vi "数据合并程序.vi"(8 "Save Files":path, 9 "File B":path, 10 "File A":path, 11 "File Item":path) -> ()   [LabVIEW 2011]
uses:
  <vilib>/Utility/file.llb/Read From Spreadsheet File (string).vi
  <vilib>/Utility/file.llb/Write To Spreadsheet File (string).vi
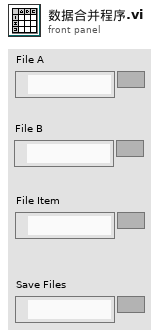
[diagram p1: front panel]
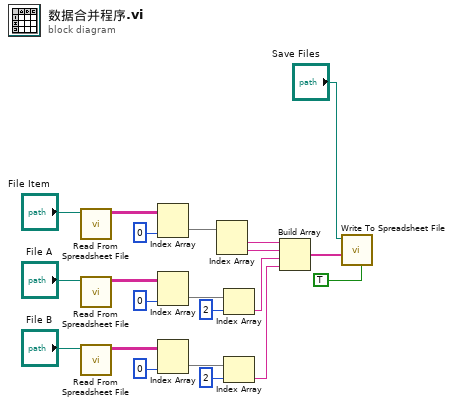
[diagram p0: block diagram]
diagram:
  n1 = call-poly <vilib>:"Read From Spreadsheet File.vi"("file path (dialog if empty)"="File Item") -> ("all rows"=w15:string[][])  [unwired: 6 in, 4 out]
  n2 = call-poly <vilib>:"Read From Spreadsheet File.vi"("file path (dialog if empty)"="File A") -> ("all rows"=w20:string[][])  [unwired: 6 in, 4 out]
  n3 = call-poly <vilib>:"Read From Spreadsheet File.vi"("file path (dialog if empty)"="File B") -> ("all rows"=w7:string[][])  [unwired: 6 in, 4 out]
  n4 = Index Array(array=w15, index (col)=0 ("禁用的索引 (列)")) -> (element=w14:string[])  [unwired: 1 in]
  n5 = Index Array(array=w20, index (col)=0 ("禁用的索引 (列)")) -> (element=w18:string[])  [unwired: 1 in]
  n6 = Index Array(array=w7, index (col)=0 ("禁用的索引 (列)")) -> (element=w11:string[])  [unwired: 1 in]
  n7 = Index Array(array=w14) -> (element #1=w6:string, element #2=w5:string)  [unwired: 2 in]
  n8 = Index Array(array=w18, index=2 ("索引")) -> (element=w4:string)
  n9 = Index Array(array=w11, index=2 ("索引")) -> (element=w3:string)
  n10 = Build Array(w6, w5, w4, w3) -> (w2:string[])
  n11 = call-poly <vilib>:"Write To Spreadsheet File.vi"("transpose? (no:F)"=TRUE, "1D data"=w2, "file path (dialog if empty)"="Save Files") -> ()  [unwired: 5 in, 1 out]
